vi "מחסן 8.11.vi"() -> ()   [LabVIEW 2013]
uses:
  Global 3.vi
panel:
  out "Water":dbl(slide) scale=0.0..50.0
  out "Virus B":dbl(slide) scale=0.0..80.0
  out "Virus C":dbl(slide) scale=0.0..80.0
  out "Classifier material":dbl(slide) scale=0.0..25.0
  out "Virus A":dbl(slide) scale=0.0..80.0
  in  "water fool":bool
  in  "A fool":bool
  in  "b fool":bool
  in  "c fool":bool
  in  "material fool":bool
  in  "Exit":bool
  out "Array 4":dbl[](array[numeric])
  in  "Array 2":dbl[](array[numeric])
  # "Fider - Warehouse"
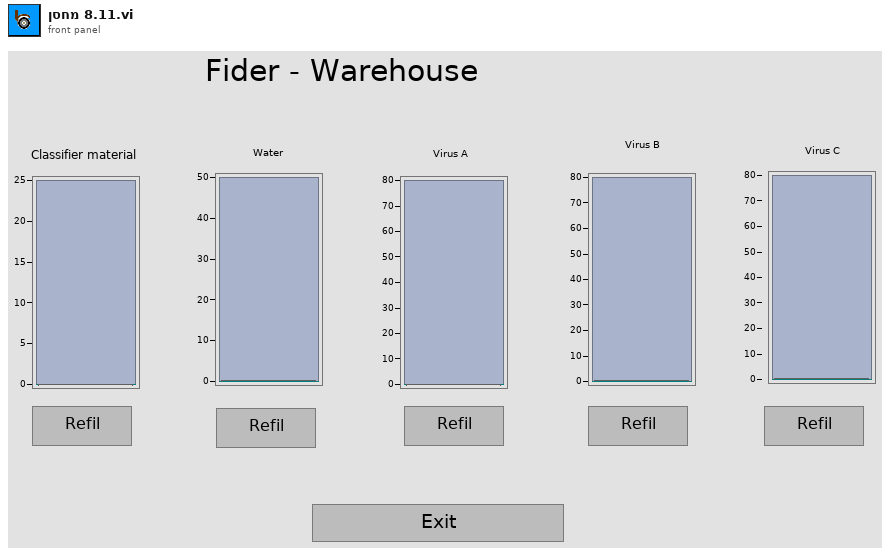
[diagram p1: front panel]
types:
  T1 = enum8{"Enabled", "Disabled", "Disabled and Grayed Out"}
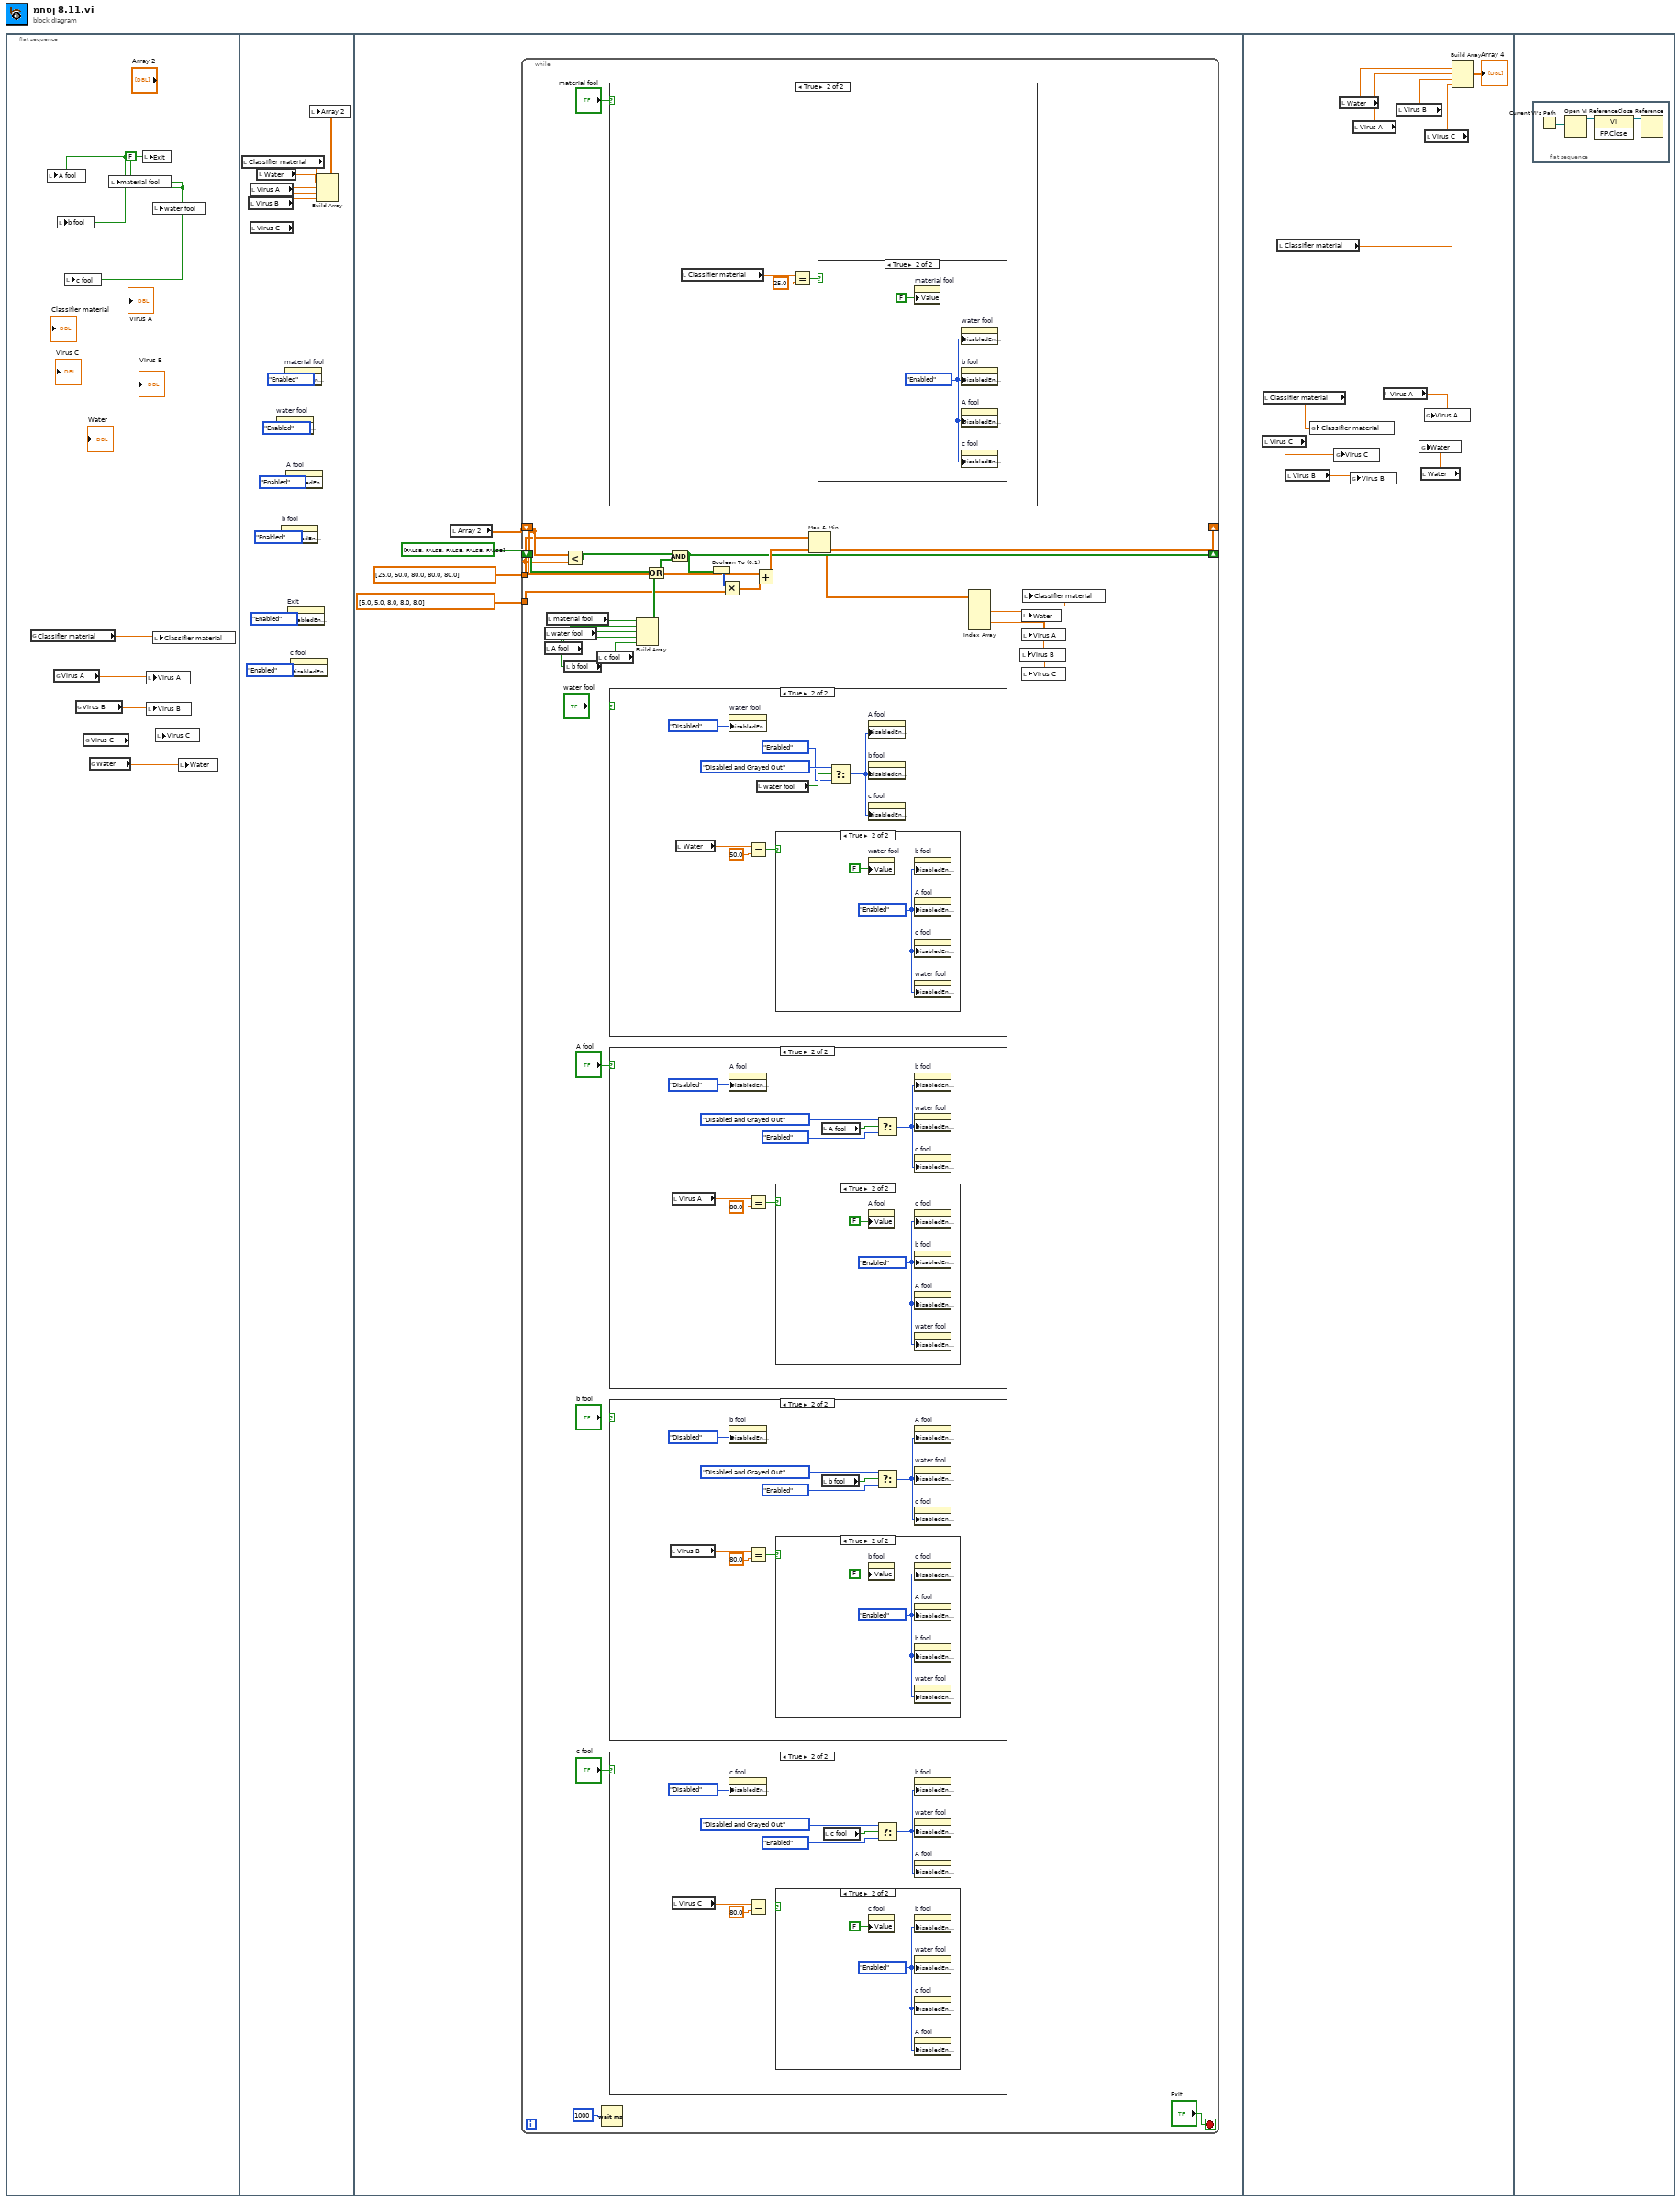
[diagram p0: block diagram]
diagram:
  n1 = flat-sequence {
    frame #0 {
      w6 = FALSE ("Exit")
      n2 = global read "Global 3.vi" "Classifier material"() -> (w5:dbl)
      n3 = local write "A fool"(w6) -> ()
      n4 = global read "Global 3.vi" "Virus A"() -> (w4:dbl)
      n5 = local write "b fool"(w6) -> ()
      n6 = local write "c fool"(w6) -> ()
      n7 = global read "Global 3.vi" "Virus B"() -> (w3:dbl)
      n8 = global read "Global 3.vi" "Virus C"() -> (w2:dbl)
      n9 = global read "Global 3.vi" "Water"() -> (w1:dbl)
      n10 = local write "material fool"(w6) -> ()
      n11 = local write "Exit"(w6) -> ()
      n12 = local write "Virus A"(w4) -> ()
      n13 = local write "Virus B"(w3) -> ()
      n14 = local write "water fool"(w6) -> ()
      n15 = local write "Classifier material"(w5) -> ()
      n16 = local write "Virus C"(w2) -> ()
      n17 = local write "Water"(w1) -> ()
    }
    frame #1 {
      n18 = local read "Classifier material"() -> (w12:dbl)
      n19 = local read "Virus B"() -> (w9:dbl)
      n20 = local read "Virus A"() -> (w10:dbl)
      n21 = local read "Virus C"() -> (w8:dbl)
      n22 = local read "Water"() -> (w11:dbl)
      n23 = property on="water fool" class="Bool (strict)"("DisabledEnum"=T1."Enabled" ("Disabled")) -> ()  [unwired: 2 in, 2 out]
      n24 = property on="b fool" class="Bool (strict)"("DisabledEnum"=T1."Enabled" ("Disabled")) -> ()  [unwired: 2 in, 2 out]
      n25 = property on="material fool" class="Bool (strict)"("DisabledEnum"=T1."Enabled" ("Disabled")) -> ()  [unwired: 2 in, 2 out]
      n26 = property on="A fool" class="Bool (strict)"("DisabledEnum"=T1."Enabled" ("Disabled")) -> ()  [unwired: 2 in, 2 out]
      n27 = property on="Exit" class="Bool (strict)"("DisabledEnum"=T1."Enabled" ("Disabled")) -> ()  [unwired: 2 in, 2 out]
      n28 = property on="c fool" class="Bool (strict)"("DisabledEnum"=T1."Enabled" ("Disabled")) -> ()  [unwired: 2 in, 2 out]
      n29 = Build Array(w12, w11, w10, w9, w8) -> (w7:dbl[])
      n30 = local write "Array 2"(w7) -> ()
    }
    frame #2 {
      n31 = local read "Array 2"() -> (w22:dbl[])
      n32 = while {
        shift-right: [w29] -> _
        shift-left: bool[] [FALSE, FALSE, FALSE, FALSE, FALSE] ("y") -> [w42]
        shift-right: [w28] -> _
        shift-left: w22 -> [w32]
        tunnel: dbl[] [25.0, 50.0, 80.0, 80.0, 80.0] ("y") -> [w30]
        tunnel: dbl[] [5.0, 5.0, 8.0, 8.0, 8.0] ("y") -> [w34]
        stop <- "Exit" stop-if-true
        n33 = local read "water fool"() -> (w40:bool)
        n34 = local read "A fool"() -> (w39:bool)
        n35 = local read "material fool"() -> (w41:bool)
        n36 = Less?(x=w32, y=w30) -> (x < y?=w44:bool[])
        n37 = local read "b fool"() -> (w38:bool)
        n38 = local read "c fool"() -> (w37:bool)
        n39 = Wait (ms)(milliseconds to wait=u32 1000) -> ()  [unwired: 1 out]
        n40 = case shown="True" "material fool" {
          frame False {
          }
          frame True {
            n41 = local read "Classifier material"() -> (w94:dbl)
            n42 = Equal?(x=w94, y=25.0) -> (x = y?=w92:bool)
            n43 = case shown="True" w92 {
              frame False {
              }
              frame True {
                w96 = T1."Enabled" ("Disabled")
                n44 = property on="material fool" class="Bool (strict)"("Value"=FALSE) -> ()  [unwired: 2 in, 2 out]
                n45 = property on="water fool" class="Bool (strict)"("DisabledEnum"=w96) -> ()  [unwired: 2 in, 2 out]
                n46 = property on="b fool" class="Bool (strict)"("DisabledEnum"=w96) -> ()  [unwired: 2 in, 2 out]
                n47 = property on="A fool" class="Bool (strict)"("DisabledEnum"=w96) -> ()  [unwired: 2 in, 2 out]
                n48 = property on="c fool" class="Bool (strict)"("DisabledEnum"=w96) -> ()  [unwired: 2 in, 2 out]
              }
            }
          }
        }
        n49 = case shown="True" "water fool" {
          frame False {
          }
          frame True {
            n50 = local read "Water"() -> (w85:dbl)
            n51 = property on="water fool" class="Bool (strict)"("DisabledEnum"=T1."Disabled" ("Disabled")) -> ()  [unwired: 2 in, 2 out]
            n52 = Equal?(x=w85, y=50.0) -> (x = y?=w83:bool)
            n53 = local read "water fool"() -> (w87:bool)
            n54 = case shown="True" w83 {
              frame False {
              }
              frame True {
                w90 = T1."Enabled" ("Disabled")
                n55 = property on="water fool" class="Bool (strict)"("Value"=FALSE) -> ()  [unwired: 2 in, 2 out]
                n56 = property on="b fool" class="Bool (strict)"("DisabledEnum"=w90) -> ()  [unwired: 2 in, 2 out]
                n57 = property on="A fool" class="Bool (strict)"("DisabledEnum"=w90) -> ()  [unwired: 2 in, 2 out]
                n58 = property on="c fool" class="Bool (strict)"("DisabledEnum"=w90) -> ()  [unwired: 2 in, 2 out]
                n59 = property on="water fool" class="Bool (strict)"("DisabledEnum"=w90) -> ()  [unwired: 2 in, 2 out]
              }
            }
            n60 = Select(t=T1."Disabled and Grayed Out" ("Disabled"), s=w87, f=T1."Enabled" ("Disabled")) -> (s? t:f=w89:T1)
            n61 = property on="A fool" class="Bool (strict)"("DisabledEnum"=w89) -> ()  [unwired: 2 in, 2 out]
            n62 = property on="b fool" class="Bool (strict)"("DisabledEnum"=w89) -> ()  [unwired: 2 in, 2 out]
            n63 = property on="c fool" class="Bool (strict)"("DisabledEnum"=w89) -> ()  [unwired: 2 in, 2 out]
          }
        }
        n64 = case shown="True" "A fool" {
          frame False {
          }
          frame True {
            n65 = local read "Virus A"() -> (w75:dbl)
            n66 = property on="A fool" class="Bool (strict)"("DisabledEnum"=T1."Disabled" ("Disabled")) -> ()  [unwired: 2 in, 2 out]
            n67 = Equal?(x=w75, y=80.0) -> (x = y?=w73:bool)
            n68 = case shown="True" w73 {
              frame False {
              }
              frame True {
                w80 = T1."Enabled" ("Disabled")
                n69 = property on="A fool" class="Bool (strict)"("Value"=FALSE) -> ()  [unwired: 2 in, 2 out]
                n70 = property on="c fool" class="Bool (strict)"("DisabledEnum"=w80) -> ()  [unwired: 2 in, 2 out]
                n71 = property on="b fool" class="Bool (strict)"("DisabledEnum"=w80) -> ()  [unwired: 2 in, 2 out]
                n72 = property on="A fool" class="Bool (strict)"("DisabledEnum"=w80) -> ()  [unwired: 2 in, 2 out]
                n73 = property on="water fool" class="Bool (strict)"("DisabledEnum"=w80) -> ()  [unwired: 2 in, 2 out]
              }
            }
            n74 = local read "A fool"() -> (w78:bool)
            n75 = Select(t=T1."Disabled and Grayed Out" ("Disabled"), s=w78, f=T1."Enabled" ("Disabled")) -> (s? t:f=w76:T1)
            n76 = property on="b fool" class="Bool (strict)"("DisabledEnum"=w76) -> ()  [unwired: 2 in, 2 out]
            n77 = property on="water fool" class="Bool (strict)"("DisabledEnum"=w76) -> ()  [unwired: 2 in, 2 out]
            n78 = property on="c fool" class="Bool (strict)"("DisabledEnum"=w76) -> ()  [unwired: 2 in, 2 out]
          }
        }
        n79 = case shown="True" "b fool" {
          frame False {
          }
          frame True {
            n80 = local read "Virus B"() -> (w64:dbl)
            n81 = property on="b fool" class="Bool (strict)"("DisabledEnum"=T1."Disabled" ("Disabled")) -> ()  [unwired: 2 in, 2 out]
            n82 = Equal?(x=w64, y=80.0) -> (x = y?=w63:bool)
            n83 = case shown="True" w63 {
              frame False {
              }
              frame True {
                w70 = T1."Enabled" ("Disabled")
                n84 = property on="b fool" class="Bool (strict)"("Value"=FALSE) -> ()  [unwired: 2 in, 2 out]
                n85 = property on="c fool" class="Bool (strict)"("DisabledEnum"=w70) -> ()  [unwired: 2 in, 2 out]
                n86 = property on="A fool" class="Bool (strict)"("DisabledEnum"=w70) -> ()  [unwired: 2 in, 2 out]
                n87 = property on="b fool" class="Bool (strict)"("DisabledEnum"=w70) -> ()  [unwired: 2 in, 2 out]
                n88 = property on="water fool" class="Bool (strict)"("DisabledEnum"=w70) -> ()  [unwired: 2 in, 2 out]
              }
            }
            n89 = local read "b fool"() -> (w67:bool)
            n90 = Select(t=T1."Disabled and Grayed Out" ("Disabled"), s=w67, f=T1."Enabled" ("Disabled")) -> (s? t:f=w69:T1)
            n91 = property on="A fool" class="Bool (strict)"("DisabledEnum"=w69) -> ()  [unwired: 2 in, 2 out]
            n92 = property on="water fool" class="Bool (strict)"("DisabledEnum"=w69) -> ()  [unwired: 2 in, 2 out]
            n93 = property on="c fool" class="Bool (strict)"("DisabledEnum"=w69) -> ()  [unwired: 2 in, 2 out]
          }
        }
        n94 = case shown="True" "c fool" {
          frame False {
          }
          frame True {
            n95 = local read "Virus C"() -> (w57:dbl)
            n96 = property on="c fool" class="Bool (strict)"("DisabledEnum"=T1."Disabled" ("Disabled")) -> ()  [unwired: 2 in, 2 out]
            n97 = Equal?(x=w57, y=80.0) -> (x = y?=w58:bool)
            n98 = case shown="True" w58 {
              frame False {
              }
              frame True {
                w60 = T1."Enabled" ("Disabled")
                n99 = property on="c fool" class="Bool (strict)"("Value"=FALSE) -> ()  [unwired: 2 in, 2 out]
                n100 = property on="b fool" class="Bool (strict)"("DisabledEnum"=w60) -> ()  [unwired: 2 in, 2 out]
                n101 = property on="water fool" class="Bool (strict)"("DisabledEnum"=w60) -> ()  [unwired: 2 in, 2 out]
                n102 = property on="c fool" class="Bool (strict)"("DisabledEnum"=w60) -> ()  [unwired: 2 in, 2 out]
                n103 = property on="A fool" class="Bool (strict)"("DisabledEnum"=w60) -> ()  [unwired: 2 in, 2 out]
              }
            }
            n104 = local read "c fool"() -> (w54:bool)
            n105 = Select(t=T1."Disabled and Grayed Out" ("Disabled"), s=w54, f=T1."Enabled" ("Disabled")) -> (s? t:f=w56:T1)
            n106 = property on="b fool" class="Bool (strict)"("DisabledEnum"=w56) -> ()  [unwired: 2 in, 2 out]
            n107 = property on="water fool" class="Bool (strict)"("DisabledEnum"=w56) -> ()  [unwired: 2 in, 2 out]
            n108 = property on="A fool" class="Bool (strict)"("DisabledEnum"=w56) -> ()  [unwired: 2 in, 2 out]
          }
        }
        n109 = Build Array(w41, w40, w39, w38, w37) -> (w36:bool[])
        n110 = Or(x=w42, y=w36) -> (x .or. y?=w43:bool[])
        n111 = And(x=w44, y=w43) -> (x .and. y?=w29:bool[])
        n112 = Boolean To (0,1)(Boolean=w29) -> (0, 1=w35:i16[])
        n113 = Multiply(x=w35, y=w34) -> (x*y=w33:dbl[])
        n114 = Add(x=w32, y=w33) -> (x+y=w31:dbl[])
        n115 = Max & Min(x=w30, y=w31) -> (min(x,y)=w28:dbl[])  [unwired: 1 out]
        n116 = Index Array(array=w28) -> (element #1=w27:dbl, element #2=w26:dbl, element #3=w25:dbl, element #4=w24:dbl, element #5=w23:dbl)  [unwired: 5 in]
        n117 = local write "Virus B"(w24) -> ()
        n118 = local write "Water"(w26) -> ()
        n119 = local write "Virus A"(w25) -> ()
        n120 = local write "Virus C"(w23) -> ()
        n121 = local write "Classifier material"(w27) -> ()
      }
    }
    frame #3 {
      n122 = local read "Virus C"() -> (w100:dbl)
      n123 = local read "Classifier material"() -> (w101:dbl)
      n124 = local read "Classifier material"() -> (w102:dbl)
      n125 = local read "Virus B"() -> (w99:dbl)
      n126 = global write "Global 3.vi" "Classifier material"(w101) -> ()
      n127 = global write "Global 3.vi" "Virus C"(w100) -> ()
      n128 = local read "Water"() -> (w107:dbl)
      n129 = global write "Global 3.vi" "Virus B"(w99) -> ()
      n130 = local read "Virus A"() -> (w106:dbl)
      n131 = local read "Virus A"() -> (w98:dbl)
      n132 = local read "Virus B"() -> (w105:dbl)
      n133 = local read "Water"() -> (w97:dbl)
      n134 = global write "Global 3.vi" "Water"(w97) -> ()
      n135 = global write "Global 3.vi" "Virus A"(w98) -> ()
      n136 = local read "Virus C"() -> (w104:dbl)
      n137 = Build Array(w102, w107, w106, w105, w104) -> (→"Array 4":dbl[])
    }
    frame #4 {
      n138 = flat-sequence {
        frame #0 {
          n139 = Current VI's Path() -> (path=w110:path)
          n140 = Open VI Reference(vi path=w110) -> (vi reference=w109:refnum<vi>)  [unwired: 5 in, 1 out]
          n141 = invoke class="VI" method="FP.Close"(reference=w109) -> (reference out=w108:refnum<vi>)  [unwired: 2 in, 2 out]
          n142 = Close Reference(reference=w108) -> ()  [unwired: 1 in, 1 out]
        }
      }
    }
  }
